vi "Directory.vi"() -> ()   [LabVIEW 2010]
uses:
  lib/Snap7.lvlib
panel:
  out "?":string
  out "Status":string
  out "Count":i32
  out "List":u16[](array[numeric])
  in  "stop":bool
  in  "BlockType":i32(ring)=65 items=["OB"=56, "DB"=65, "SDB"=66, "FC"=67, "SFC"=68, "FB"=69, "SFB"=70]
  out "BlockList":T1
  in  "Slot":i32=2
  in  "Rack":i32
  in  "Address IP":string="192.168.1.12"
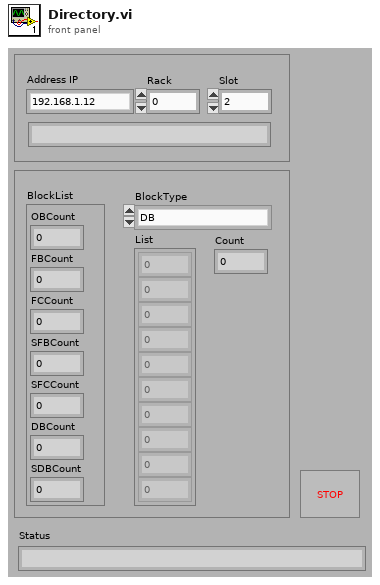
[diagram p1: front panel]
types:
  T1 = cluster{"OBCount":i32, "FBCount":i32, "FCCount":i32, "SFBCount":i32, "SFCCount":i32, "DBCount":i32, "SDBCount":i32}
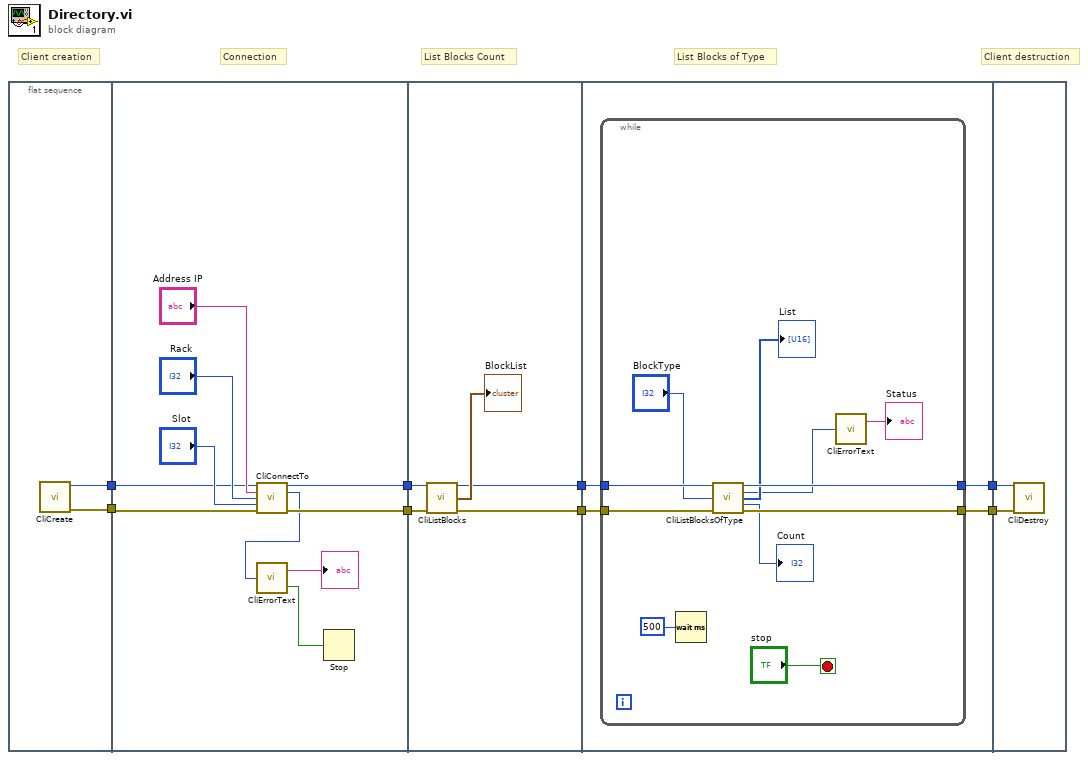
[diagram p0: block diagram]
diagram:
  # "List Blocks Count"
  # "List Blocks of Type"
  # "Client destruction"
  # "Connection"
  # "Client creation"
  n1 = flat-sequence {
    tunnel: [w10] -> w6
    tunnel: [w9] -> w5
    tunnel: [w20] -> w8
    tunnel: [w14] -> w7
    tunnel: w6 -> [w16]
    tunnel: w5 -> [w15]
    tunnel: w8 -> [w24]
    tunnel: w7 -> [w25]
    tunnel: [w22] -> w4
    tunnel: [w21] -> w3
    tunnel: [w29] -> w2
    tunnel: w3 -> [w27]
    tunnel: w4 -> [w28]
    tunnel: [w26] -> w1
    tunnel: w2 -> [w42]
    tunnel: w1 -> [w41]
    frame #0 {
      n2 = call "CliCreate.vi"() -> ("ref out"=w10:u64, "error out"=w9:errorcluster)  [unwired: 14 in]
    }
    frame #1 {
      n3 = call "CliConnectTo.vi"("ref in"=w16, "Address"="Address IP", "Rack"="Rack", "Slot"="Slot", "error in (no error)"=w15) -> ("ref out"=w14:u64, "Result"=w11:i32, "error out"=w20:errorcluster)  [unwired: 8 in]
      n4 = call "CliErrorText.vi"("ErrNo"=w11) -> ("Error"=w12:bool, "ErrMessage"=→"?":string)
      n5 = Stop(stop? (T)=w12) -> ()
    }
    frame #2 {
      n6 = call "CliListBlocks.vi"("ref in"=w25, "error in (no error)"=w24) -> ("ref out"=w22:u64, "BlockList"=→"BlockList":T1, "error out"=w21:errorcluster)  [unwired: 10 in, 1 out]
    }
    frame #3 {
      n7 = while {
        tunnel: w28 -> [w40]
        tunnel: w27 -> [w37]
        tunnel: [w36] -> w29
        tunnel: [w35] -> w26
        stop <- "stop" stop-if-true
        n8 = Wait (ms)(milliseconds to wait=u32 500 ("Loop Delay (ms)")) -> ()  [unwired: 1 out]
        n9 = call "CliListBlocksOfType.vi"("ref in"=w40, "BlockType"="BlockType", "error in (no error)"=w37) -> ("ref out"=w36:u64, "Result"=w32:i32, "BlockList"=→"List":u16[], "ItemsCount"=→"Count":i32, "error out"=w35:errorcluster)  [unwired: 8 in]
        n10 = call "CliErrorText.vi"("ErrNo"=w32) -> ("ErrMessage"=→"Status":string)  [unwired: 1 out]
      }
    }
    frame #4 {
      n11 = call "CliDestroy.vi"("ref in"=w42, "error in (no error)"=w41) -> ()  [unwired: 13 in, 1 out]
    }
  }
